vi "Query Configuration.vi"(0 "instrument handle":refnum<k15>, 5 "StepIndex":i32 format="%.0g", 7 "WaveformBufferSize":i32=2048, 11 "error in (no error)":errorcluster {"code" format="%.0x"}) -> (1 "Time":dbl, 2 "Waveform":string, 3 "Frequency":dbl, 4 "instrument handle out":refnum<k15>, 6 "TriggerType":i32, 8 "TransitionTime":dbl, 9 "Count":i32, 10 "RadioBand":i32, 12 "StepDuration":i32, 13 "Amplitude":dbl, 14 "Link":i32, 15 "error out":errorcluster {"code" format="%.0x"})   [LabVIEW 2009, in "Keysight XSAn.lvlib"]
doc: "Query the Configuration of the List Sequencer.\n\nSupported Models: M8920A, M9420A, M9421A."
uses:
  <instrlib>/Keysight XSAn/Keysight XSAn.lvlib
  AgXSAn.dll
panel:
  out "OutputTriggerEnabled":bool
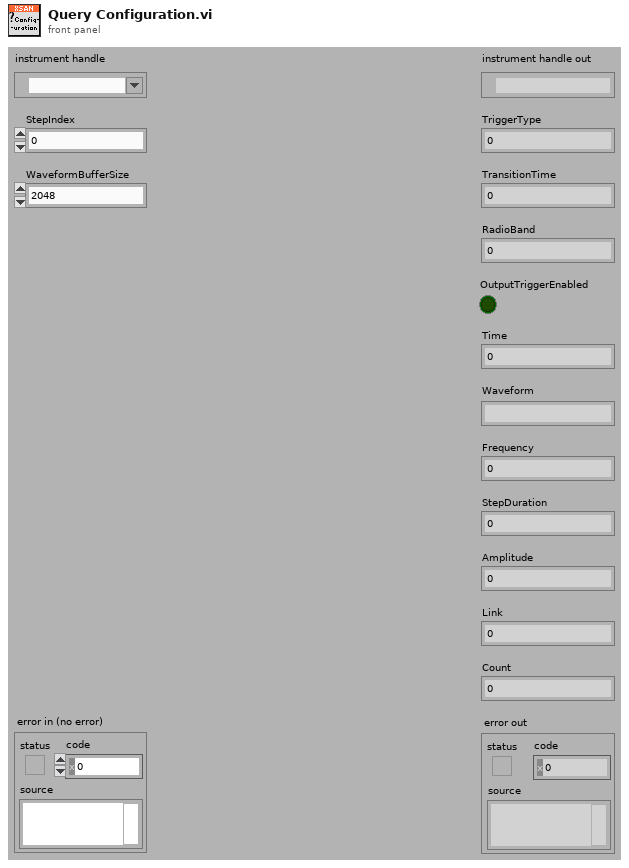
[diagram p1: front panel]
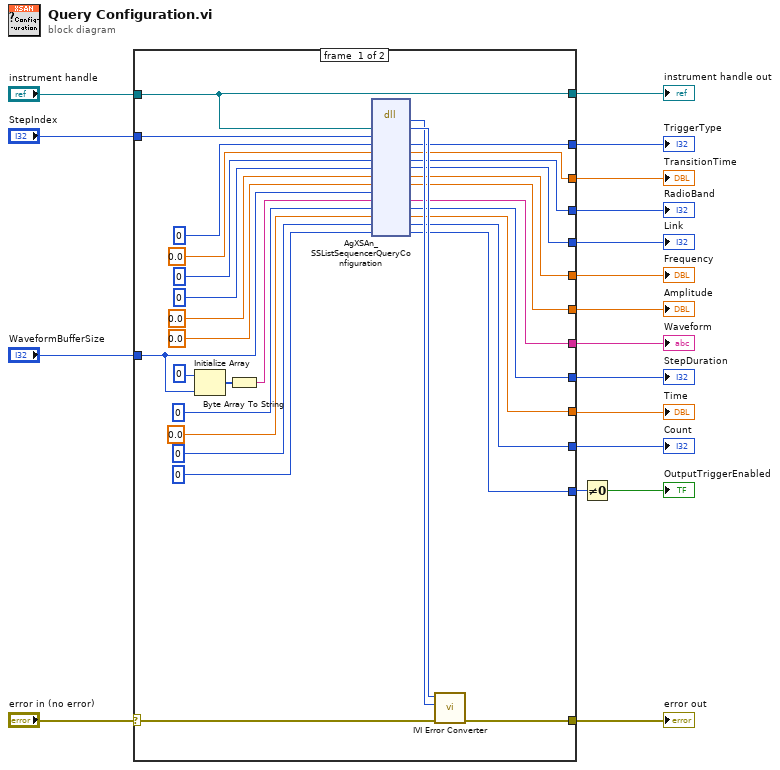
[diagram p0: block diagram]
diagram:
  n1 = case shown="No Error" "error in (no error)" {
    selector: "error in (no error)" -> [w47 w51]
    tunnel: [w46 w51] -> w18
    tunnel: "instrument handle" -> [w21 w50]
    tunnel: "StepIndex" -> [w45 _]
    tunnel: [w43 _] -> w14
    tunnel: [w41 _] -> w13
    tunnel: [w39 _] -> w12
    tunnel: [w37 _] -> w11
    tunnel: [w35 _] -> w10
    tunnel: [w33 _] -> w9
    tunnel: "WaveformBufferSize" -> [w19 _]
    tunnel: [w29 _] -> w7
    tunnel: [w27 _] -> w6
    tunnel: [w20 _] -> w5
    tunnel: [w24 _] -> w4
    tunnel: [w22 _] -> w2
    tunnel: [w21 w50] -> w1
    frame #0 {
      n2 = Initialize Array(u8 0 ("element"), w19) -> (w31:u8[])
      n3 = Byte Array To String(unsigned byte array=w31) -> (string=w32:string)
      n4 = dll-call lib="AgXSAn**.dll" fn="AgXSAn_SSListSequencerQueryConfiguration"("Vi"=w21, "StepIndex"=w45, "TriggerType"=0, "TransitionTime"=0.0, "RadioBand"=0, "Link"=0, "Frequency"=0.0, "Amplitude"=0.0, "WaveformBufferSize"=w19, "Waveform"=w32, "StepDuration"=0, "Time"=0.0, "Count"=0, "OutputTriggerEnabled"=i16 0) -> (w48:i32, "Vi"=w49:u32, "TriggerType"=w43:i32, "TransitionTime"=w41:dbl, "RadioBand"=w39:i32, "Link"=w37:i32, "Frequency"=w35:dbl, "Amplitude"=w33:dbl, "Waveform"=w29:string, "StepDuration"=w27:i32, "Time"=w20:dbl, "Count"=w24:i32, "OutputTriggerEnabled"=w22:i16)  [unwired: 5 in, 2 out]
      n5 = call <instrlib>:"IVI Error Converter.vi"("error in (no error)"=w47, "IVI error code (0)"=w48, "instrument handle"=w49) -> ("error out"=w46:errorcluster)  [unwired: 7 in, 1 out]
    }
    frame #1 {
    }
  }
  "error out" <- w18
  "instrument handle out" <- w1
  "TriggerType" <- w14
  "TransitionTime" <- w13
  "RadioBand" <- w12
  "Link" <- w11
  "Frequency" <- w10
  "Amplitude" <- w9
  "Waveform" <- w7
  "StepDuration" <- w6
  "Time" <- w5
  "Count" <- w4
  n6 = Not Equal To 0?(x=w2) -> (x != 0?=→"OutputTriggerEnabled":bool)
